vi "testXYGraph.vi"() -> ()   [LabVIEW 2019]
panel:
  out "Random index":i32[](array[numeric])=[4, 16, 17, 14, 92, 29, 8, 31, 42, 104, 84, 28, 85, 90, 13, 60, 120, 41, 111, 82, 69, 34, 7, 77, 47, 59, 65, 116, 24, 30, 113, 2, 63, 94, 106, 103, 71, 100, 22, 18, 32, 102, 19, 97, 44, 12, 0, 1, 109, 27, 88, 99, 51, 107, 76, 56, 81, 96, 72, 93, 74, 21, 5, 79, 9, 117, 38, 45, 25, 58, 105, 57, 40, 52, 23, 87, 89, 62, 26, 110, 37, 3, 101, 10, 54, 61, 83, 46, 86, 66, 68, 43, 108, 11, 67, 75, 6, 80, 49, 20, 112, 78, 115, 119, 95, 64, 73, 39, 15, 48, 55, 70, 50, 98, 91, 35, 53, 36, 118, 33, 114]
  in  "X size":dbl=11.0
  in  "Y size":dbl=11.0
  in  "XYPositions":dbl[][](array[numeric])=[[-0.09999999999999998, -0.3], [-0.09999999999999998, -0.19999999999999996], [-0.3, 0.4], [0.20000000000000007, -0.09999999999999998], [-0.5, -0.5], [0.0, 0.20000000000000007], [0.30000000000000004, 0.30000000000000004], [-0.3, -0.5], [-0.5, 0.10000000000000009], [0.0, 0.4], [0.20000000000000007, 0.10000000000000009], [0.30000000000000004, 0.0], [-0.09999999999999998, -0.4], [-0.4, -0.19999999999999996], [-0.5, -0.19999999999999996], [0.4, 0.4], [-0.5, -0.4], [-0.5, -0.3], [-0.19999999999999996, 0.10000000000000009], [-0.19999999999999996, 0.4], [0.4, -0.5], [0.0, 0.10000000000000009], [-0.19999999999999996, 0.0], [0.10000000000000009, 0.30000000000000004], [-0.3, 0.10000000000000009], [0.10000000000000009, -0.3], [0.20000000000000007, -0.4], [-0.09999999999999998, 0.0], [-0.4, -0.5], [-0.5, 0.0], [-0.3, 0.20000000000000007], [-0.5, 0.20000000000000007], [-0.19999999999999996, 0.20000000000000007], [0.5, 0.4], [-0.4, 0.5], [0.5, 0.0], [0.5, 0.20000000000000007], [0.20000000000000007, -0.19999999999999996], [0.10000000000000009, -0.5], [0.4, 0.30000000000000004], [0.10000000000000009, 0.10000000000000009], [-0.4, 0.10000000000000009], [-0.5, 0.30000000000000004], [0.30000000000000004, -0.19999999999999996], [-0.09999999999999998, -0.5], [0.10000000000000009, -0.4], [0.20000000000000007, 0.5], [-0.3, -0.3], [0.4, 0.5], [0.30000000000000004, 0.5], [0.5, -0.3], [-0.09999999999999998, 0.30000000000000004], [0.10000000000000009, 0.20000000000000007], [0.5, 0.10000000000000009], [0.20000000000000007, 0.20000000000000007], [0.5, -0.5], [0.0, -0.5], [0.10000000000000009, 0.0], [0.10000000000000009, -0.19999999999999996], [-0.3, -0.19999999999999996], [-0.4, -0.09999999999999998], [0.20000000000000007, 0.30000000000000004], [0.20000000000000007, -0.5], [-0.3, 0.5], [0.4, 0.10000000000000009], [-0.3, -0.09999999999999998], [0.30000000000000004, -0.4], [0.30000000000000004, 0.10000000000000009], [0.30000000000000004, -0.3], [-0.4, 0.4], [0.5, -0.4], [-0.19999999999999996, -0.19999999999999996], [0.0, -0.19999999999999996], [0.4, 0.20000000000000007], [0.0, 0.0], [0.30000000000000004, 0.20000000000000007], [-0.09999999999999998, 0.5], [-0.3, -0.4], [0.4, -0.3], [0.0, 0.30000000000000004], [0.30000000000000004, 0.4], [0.0, -0.4], [-0.4, 0.30000000000000004], [0.20000000000000007, 0.4], [-0.5, 0.5], [-0.4, -0.4], [0.30000000000000004, -0.5], [0.10000000000000009, 0.4], [-0.09999999999999998, 0.10000000000000009], [0.10000000000000009, 0.5], [-0.4, -0.3], [0.5, -0.09999999999999998], [-0.5, -0.09999999999999998], [0.0, -0.09999999999999998], [-0.19999999999999996, -0.5], [0.4, 0.0], [0.0, -0.3], [-0.19999999999999996, 0.5], [0.5, -0.19999999999999996], [-0.09999999999999998, 0.20000000000000007], [-0.19999999999999996, -0.09999999999999998], [0.20000000000000007, 0.0], [-0.19999999999999996, 0.30000000000000004], [-0.19999999999999996, -0.3], [-0.5, 0.4], [0.10000000000000009, -0.09999999999999998], [-0.19999999999999996, -0.4], [-0.09999999999999998, 0.4], [0.30000000000000004, -0.09999999999999998], [-0.09999999999999998, -0.09999999999999998], [0.20000000000000007, -0.3], [-0.4, 0.20000000000000007], [0.4, -0.4], [-0.3, 0.30000000000000004], [0.5, 0.5], [0.4, -0.19999999999999996], [-0.3, 0.0], [0.0, 0.5], [0.5, 0.30000000000000004], [0.4, -0.09999999999999998], [-0.4, 0.0]]
  out "XY Intensity Map":dbl[][](graph)=[[3.904687043201515e-13, 6.684989195773002e-11, 3.649880430807626e-09, 6.355065252727497e-08, 3.5287820878809013e-07, 6.248749509463085e-07, 3.5287820878809013e-07, 6.355065252727497e-08, 3.649880430807626e-09, 6.684989195773002e-11, 3.904687043201515e-13], [6.684989195773002e-11, 1.1444983952148092e-08, 6.248749509463097e-07, 1.0880140221963334e-05, 6.041424029819161e-05, 0.0001069812317752422, 6.041424029819161e-05, 1.0880140221963334e-05, 6.248749509463097e-07, 1.1444983952148092e-08, 6.684989195773002e-11], [3.649880430807626e-09, 6.248749509463097e-07, 3.41170163237202e-05, 0.0005940355282204004, 0.003298505755939091, 0.005840977343195246, 0.003298505755939091, 0.0005940355282204004, 3.41170163237202e-05, 6.248749509463097e-07, 3.649880430807626e-09], [6.355065252727497e-08, 1.0880140221963334e-05, 0.0005940355282204004, 0.01034317319661825, 0.05743261926761737, 0.10170139230422684, 0.05743261926761737, 0.01034317319661825, 0.0005940355282204004, 1.0880140221963334e-05, 6.355065252727497e-08], [3.5287820878809013e-07, 6.041424029819161e-05, 0.003298505755939091, 0.05743261926761737, 0.31890655732397044, 0.5647181220077593, 0.31890655732397044, 0.05743261926761737, 0.003298505755939091, 6.041424029819161e-05, 3.5287820878809013e-07], [6.248749509463085e-07, 0.0001069812317752422, 0.005840977343195246, 0.10170139230422684, 0.5647181220077593, 1.0, 0.5647181220077593, 0.10170139230422684, 0.005840977343195246, 0.0001069812317752422, 6.248749509463085e-07], [3.5287820878809013e-07, 6.041424029819161e-05, 0.003298505755939091, 0.05743261926761737, 0.31890655732397044, 0.5647181220077593, 0.31890655732397044, 0.05743261926761737, 0.003298505755939091, 6.041424029819161e-05, 3.5287820878809013e-07], [6.355065252727497e-08, 1.0880140221963334e-05, 0.0005940355282204004, 0.01034317319661825, 0.05743261926761737, 0.10170139230422684, 0.05743261926761737, 0.01034317319661825, 0.0005940355282204004, 1.0880140221963334e-05, 6.355065252727497e-08], [3.649880430807626e-09, 6.248749509463097e-07, 3.41170163237202e-05, 0.0005940355282204004, 0.003298505755939091, 0.005840977343195246, 0.003298505755939091, 0.0005940355282204004, 3.41170163237202e-05, 6.248749509463097e-07, 3.649880430807626e-09], [6.684989195773002e-11, 1.1444983952148092e-08, 6.248749509463097e-07, 1.0880140221963334e-05, 6.041424029819161e-05, 0.0001069812317752422, 6.041424029819161e-05, 1.0880140221963334e-05, 6.248749509463097e-07, 1.1444983952148092e-08, 6.684989195773002e-11], [3.904687043201515e-13, 6.684989195773002e-11, 3.649880430807626e-09, 6.355065252727497e-08, 3.5287820878809013e-07, 6.248749509463085e-07, 3.5287820878809013e-07, 6.355065252727497e-08, 3.649880430807626e-09, 6.684989195773002e-11, 3.904687043201515e-13]]
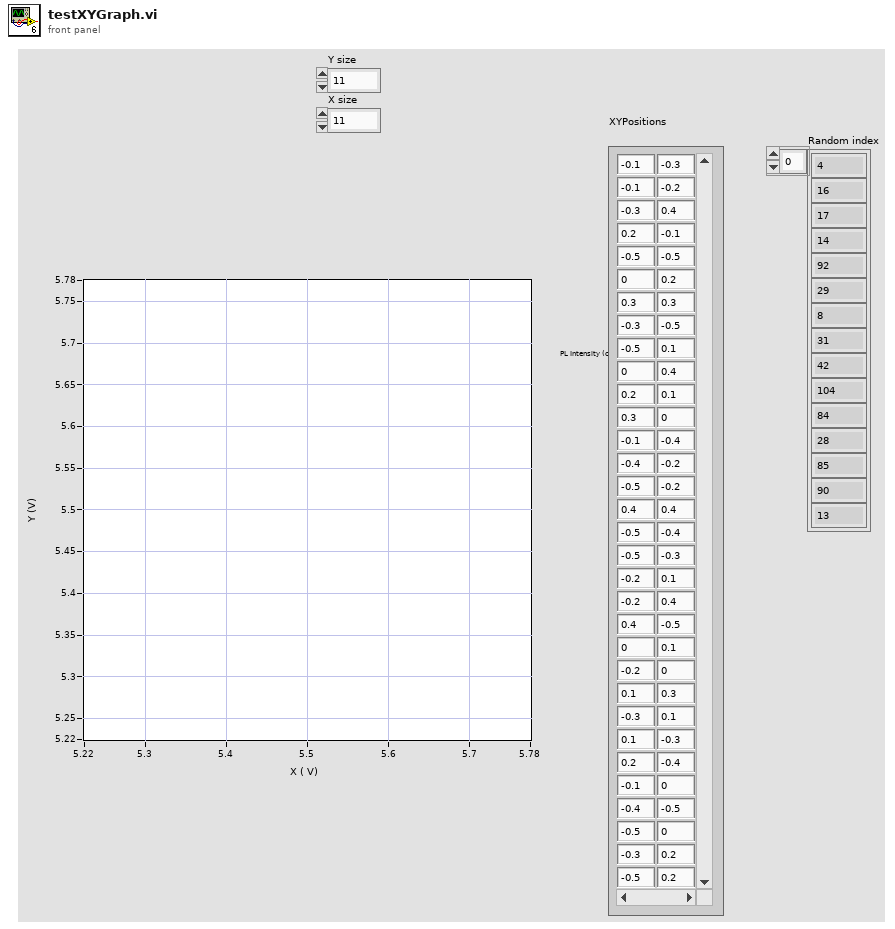
[diagram p1: front panel]
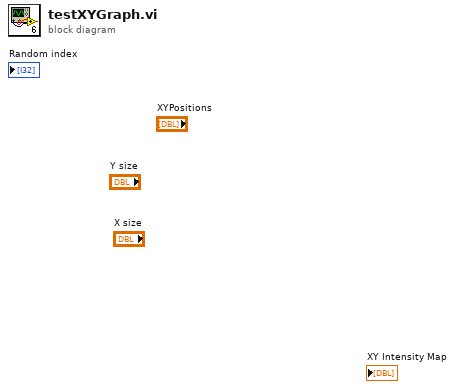
[diagram p0: block diagram]
diagram:
